vi "Manipulator Panel.vi"() -> ()   [LabVIEW 2014]
uses:
  <vilib>/Platform/TimedLoop/XDataNode/timing_clust.ctl
  <vilib>/Platform/TimedLoop/XDataNode/nitl_modes.ctl
  <vilib>/Platform/TimedLoop/XDataNode/wakeup.ctl
  <vilib>/Utility/inputDevices.llb/joystickAcquire.vi
  <vilib>/Platform/TimedLoop/XDataNode/XDataNode.xnode
  <vilib>/Platform/TimedLoop/XDataNode/XDNodeRunTimeDep.lvlib
panel:
  in  "Joystick Selector":u16(ring) items=["HID Dongle", "USB PnP Sound Device"]
  in  "Use Joystick":bool
  out "axis info":T1
  out "button info":T2
  out "Active":bool
  out "Reset":bool
  in  "TCPConRef":refnum<k5>
  out "Turning off in":dbl=10.0
  in  "Power switch\nmanipulator":bool
  in  "Arm Rotate ccw":bool
  in  "Arm Rotate cw":bool
  in  "Claw close":bool
  in  "Claw open":bool
  in  "Arm right":bool
  in  "Arm left":bool
  in  "Lower arm down":bool
  in  "Lower arm up":bool
  in  "Upper arm down":bool
  in  "Upper arm up":bool
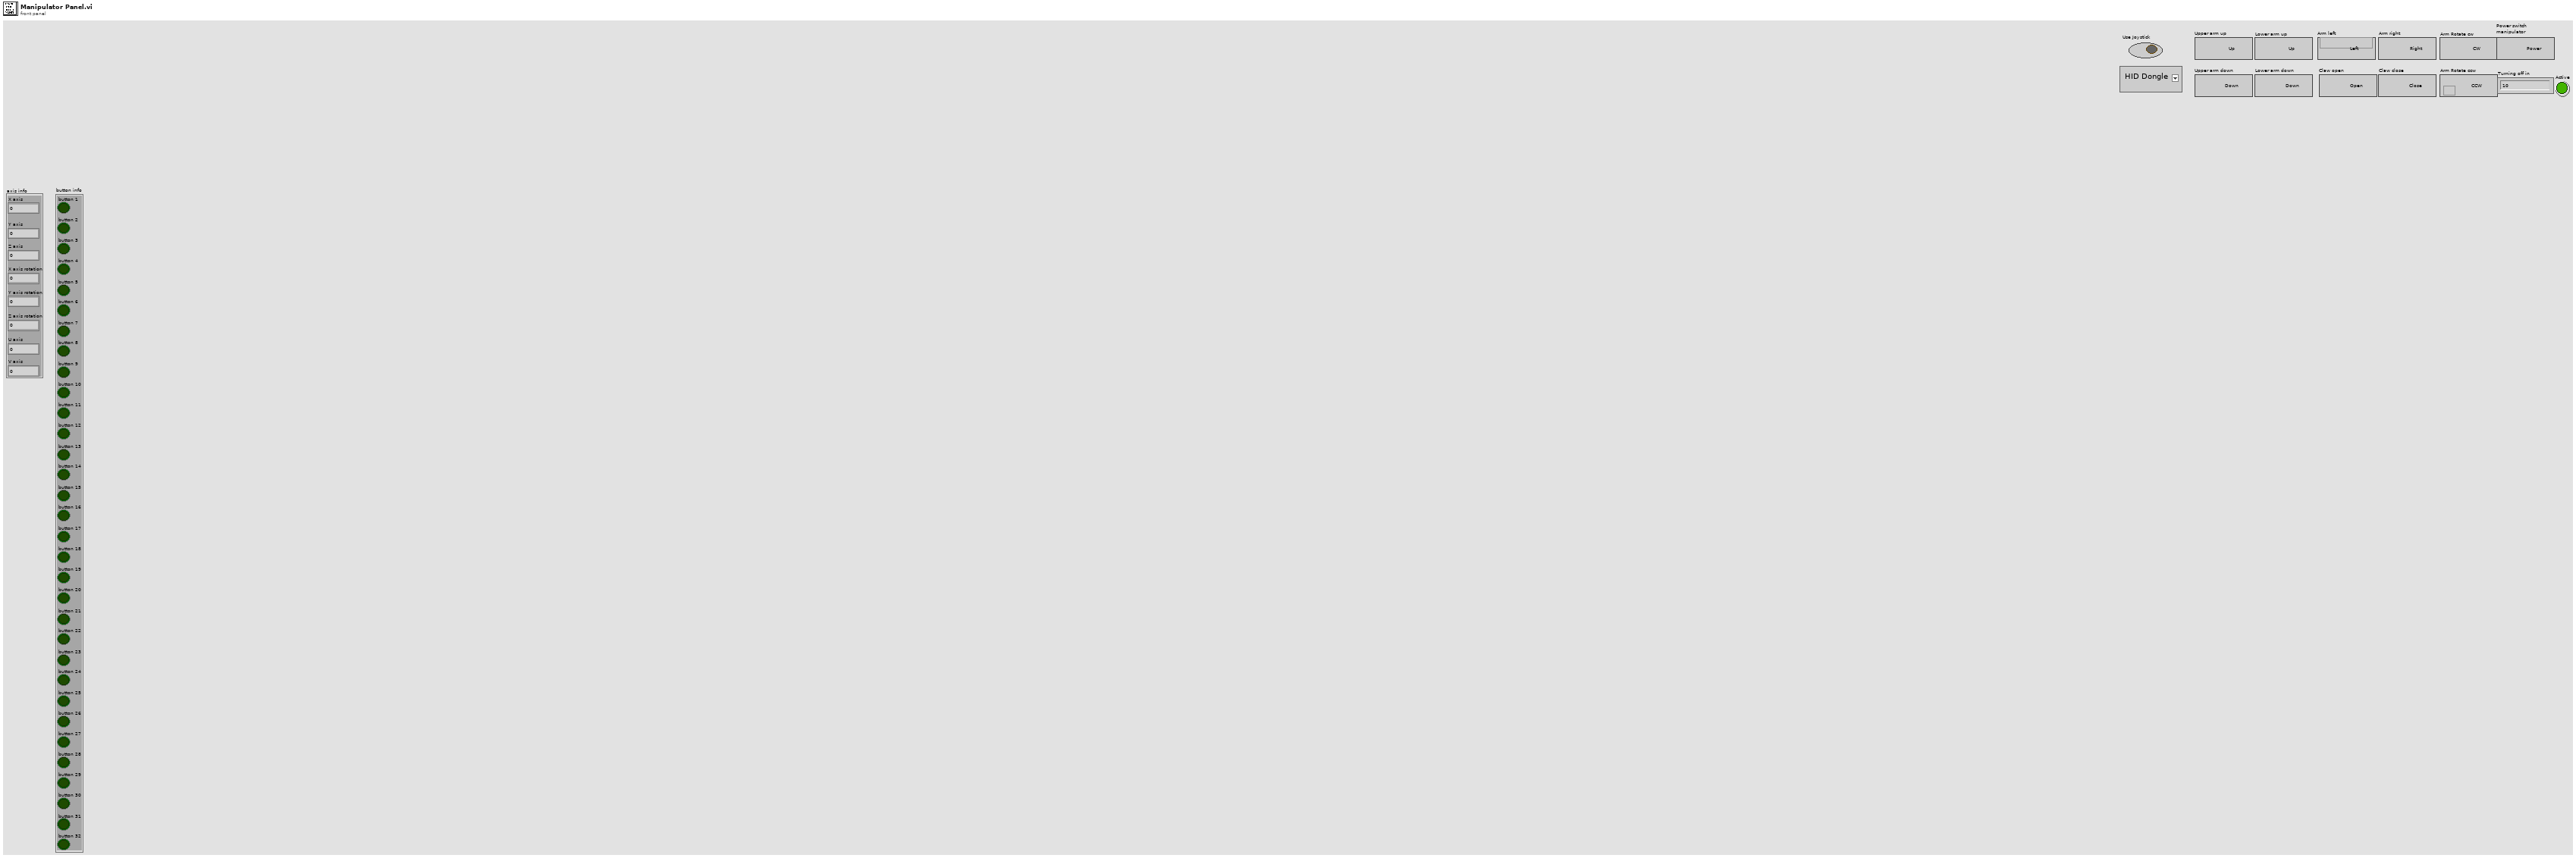
[diagram p1: front panel]
types:
  T1 = cluster{"X axis":i32, "Y axis":i32, "Z axis":i32, "X axis rotation":i32, "Y axis rotation":i32, "Z axis rotation":i32, "U axis":i32, "V axis":i32}
  T2 = cluster{"button 1":bool, "button 2":bool, "button 3":bool, "button 4":bool, "button 5":bool, "button 6":bool, "button 7":bool, "button 8":bool, "button 9":bool, "button 10":bool, "button 11":bool, "button 12":bool, "button 13":bool, "button 14":bool, "button 15":bool, "button 16":bool, "button 17":bool, "button 18":bool, "button 19":bool, "button 20":bool, "button 21":bool, "button 22":bool, "button 23":bool, "button 24":bool, "button 25":bool, "button 26":bool, "button 27":bool, "button 28":bool, "button 29":bool, "button 30":bool, "button 31":bool, "button 32":bool}
  T3 = typedef "XDNodeRunTimeDep.lvlib/timing_clust.ctl" = cluster{"Expected End [f-1]":u64, "Actual End [f-1]":u64, "Finished Late? [f-1]":bool, "Expected End [i-1]":u64, "Actual End [i-1]":u64, "Finished Late? [i-1]":bool, "Expected Start [i]":u64, "Actual Start [i]":u64, "Expected Start [f]":u64, "Actual Start [f]":u64, "Source Name":string, "Structure Name":string, "Period":i64, "Deadline":i64, "Offset":i64, "Start":i64, "Priority":i32, "Timeout":i32, "Mode":T4, "Wakeup Reason":T5, "Error":errorcluster, "Source Type":string, "Secondary Source Type":string, "Global End Time":u64, "Global Start Time":u64, "Frame Duration":u64, "Iteration Duration":u64, "Assigned CPU":i32, "I/O Scan Engine Mode":u32}
  T4 = typedef "XDNodeRunTimeDep.lvlib/nitl_modes.ctl" = enum32{"No Change", "Process missed periods, maintain original phase", "Discard missed periods, maintain original phase", "Process missed periods, ignore original phase", "Discard missed periods, ignore original phase"}
  T5 = typedef "XDNodeRunTimeDep.lvlib/wakeup.ctl" = enum32{"Normal", "Aborted", "Asynchronous wakeup", "Timing source error", "Timed loop error", "Timeout"}
  T6 = cluster{"axes total":u32, "buttons total":u32, "pov total":u32, "device name":string}[]
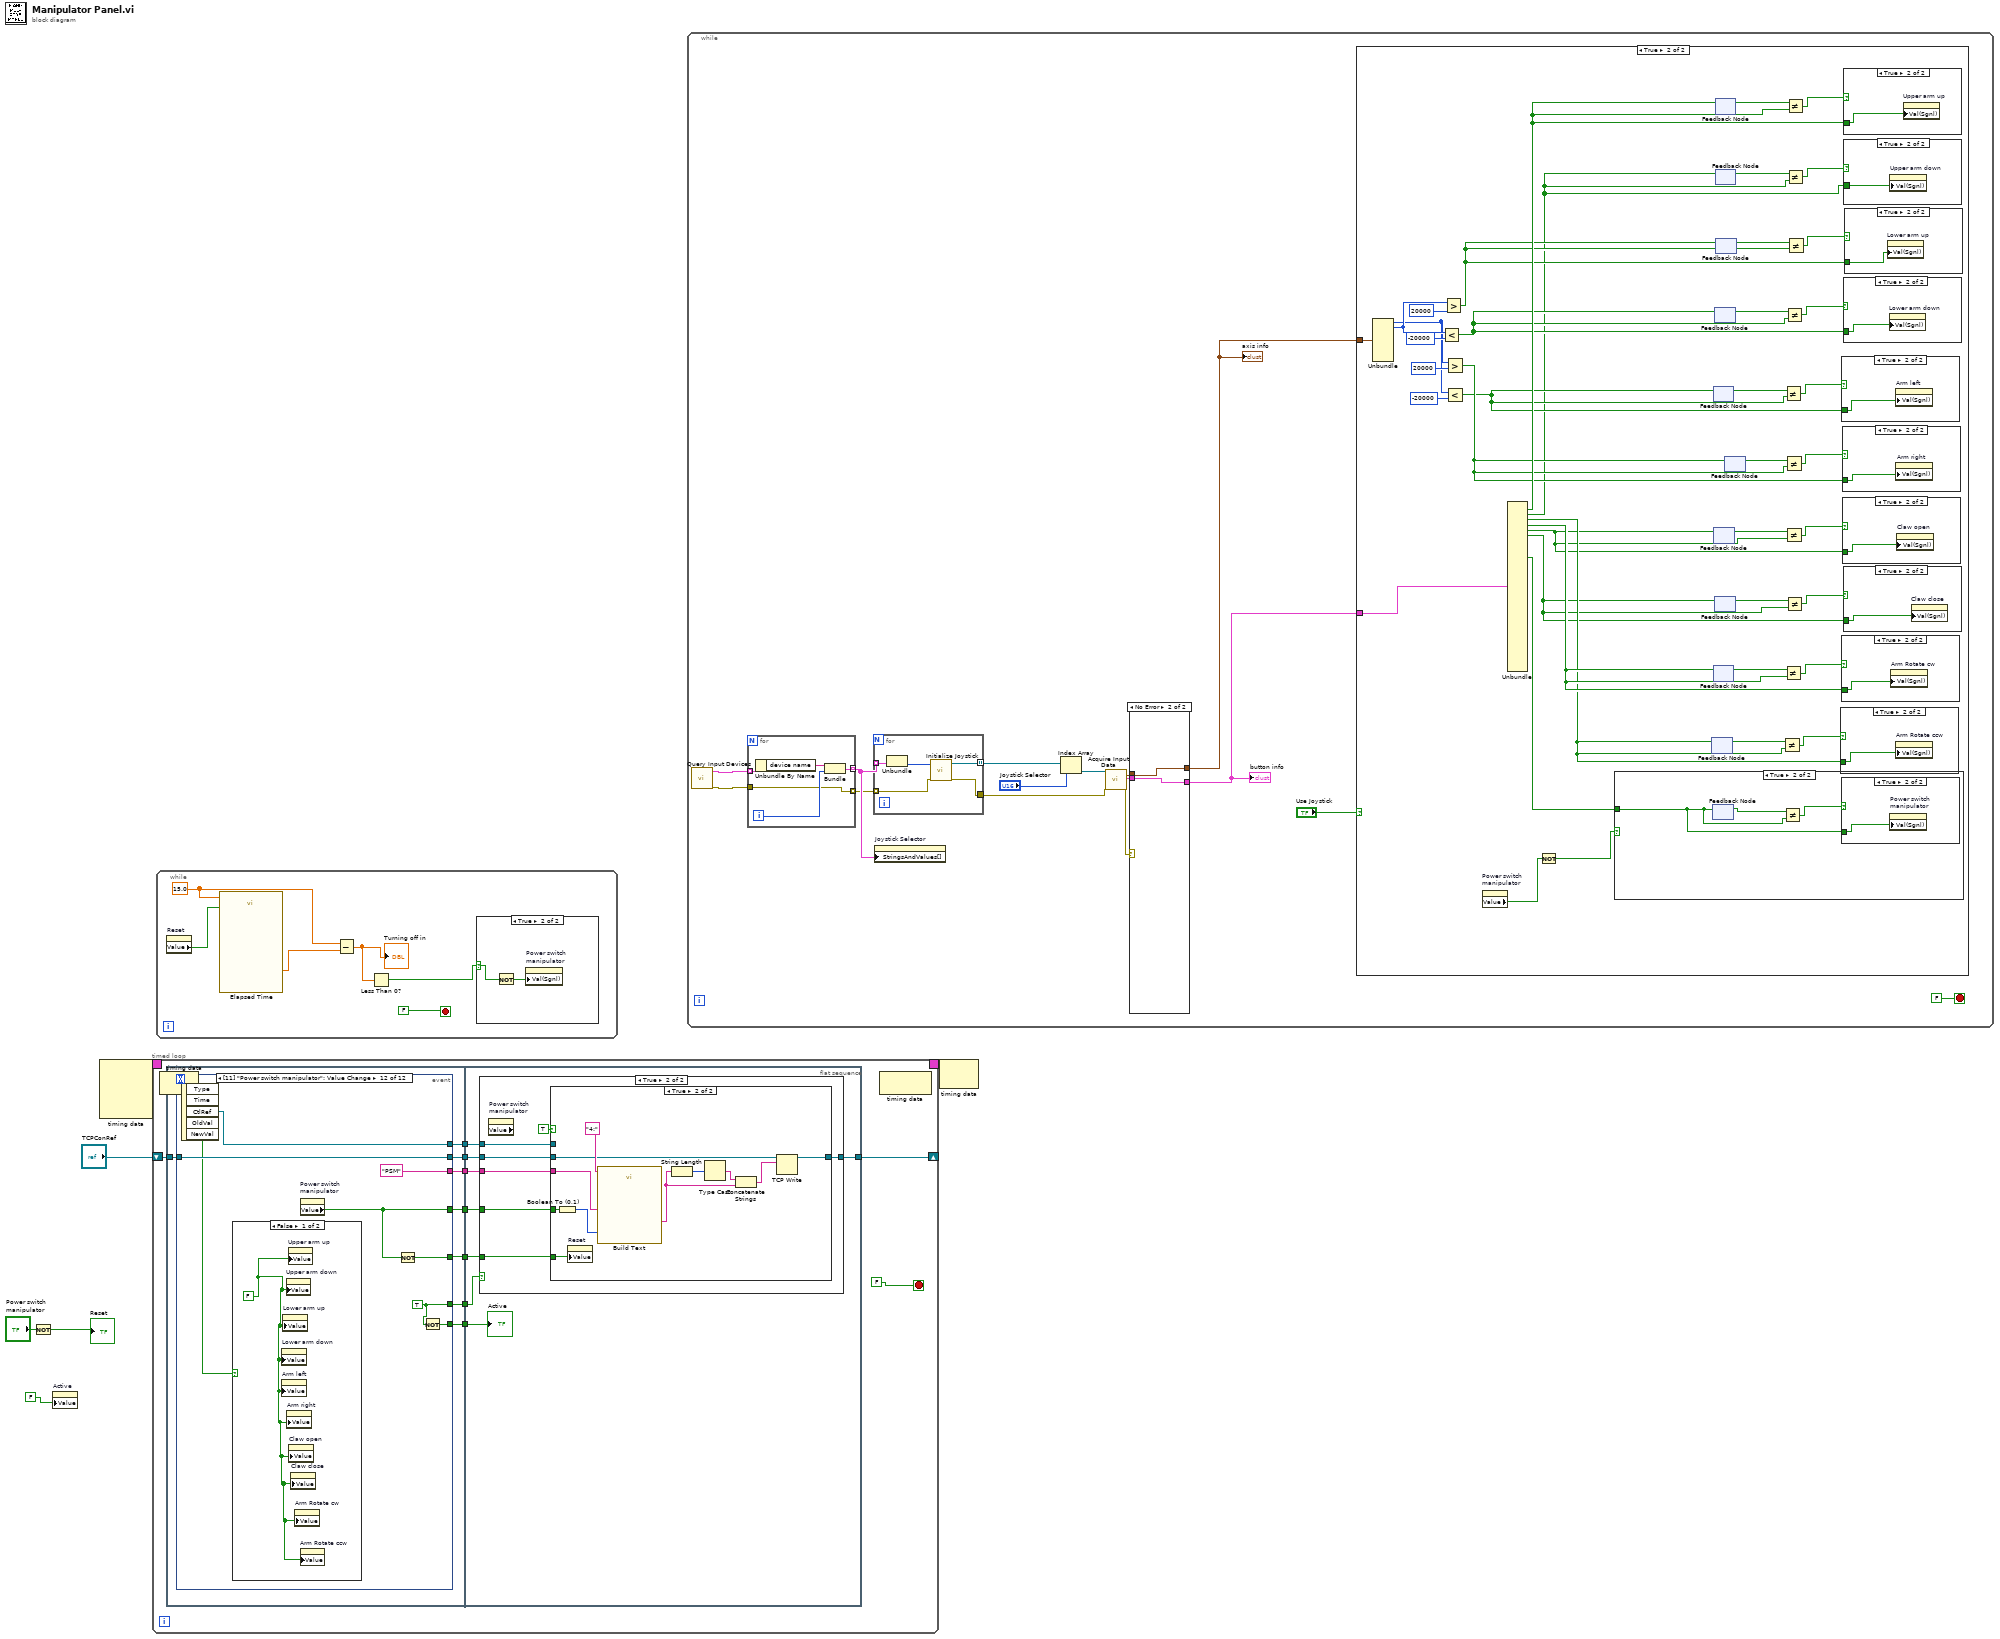
[diagram p0: block diagram]
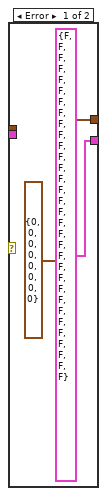
[diagram p2: hidden frame]
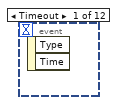
[diagram p16: hidden frame]
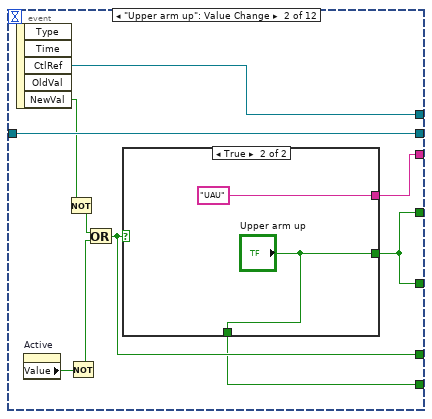
[diagram p17: hidden frame]
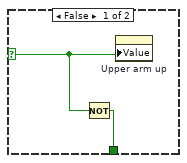
[diagram p18: hidden frame]
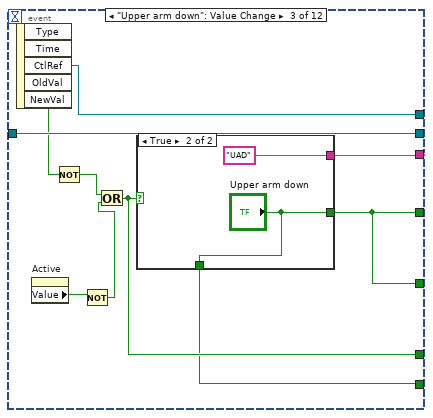
[diagram p19: hidden frame]
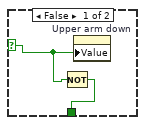
[diagram p20: hidden frame]
diagram:
  n1 = Not(x="Power switch\nmanipulator") -> (.not. x?=→"Reset":bool)
  n2 = property on="Active" class="Bool (strict)"("Value"=FALSE) -> ()  [unwired: 2 in, 2 out]
  n3 = node-c288() -> (w2:T3)  [unwired: 4 in]
  n4 = timed-loop {
    shift-right: [w9] -> _
    shift-left: "TCPConRef" -> [w15]
    timing: w2 -> [_]
    timing-out: [_] -> w1
    stop <- FALSE stop-if-true
    n5 = node-c288() -> ()  [unwired: 1 in, 1 out]
    n6 = flat-sequence {
      tunnel: w15 -> [w26]
      tunnel: [w25] -> w14
      tunnel: [w24] -> w13
      tunnel: [w23] -> w12
      tunnel: [w22] -> w11
      tunnel: [w21] -> w10
      tunnel: [w20] -> w8
      tunnel: [w19] -> w7
      tunnel: w14 -> [w182]
      tunnel: w13 -> [w181]
      tunnel: w12 -> [w180]
      tunnel: w11 -> [w183]
      tunnel: w10 -> [w179]
      tunnel: [w178] -> w9
      tunnel: w8 -> [w177]
      tunnel: w7 -> [w176]
      frame #0 {
        n7 = event shown="[11] \"Power switch manipulator\": Value Change" {
          selector: _ -> [_ _ _ _ _ _ _ _ _ _ _ _]
          dyn-events: _ -> [_ _ _ _ _ _ _ _ _ _ _ _]
          timeout: _ -> [_ _ _ _ _ _ _ _ _ _ _ _]
          tunnel: w26 -> [_ w36 w49 w63 w76 w92 w104 w119 w133 w146 w160 w173]
          tunnel: [_ w36 w49 w63 w76 w92 w104 w119 w133 w146 w160 w173] -> w25
          tunnel: [_ w30 w50 w62 w78 w91 w105 w120 w134 w147 w161 "PSM"] -> w24
          tunnel: [_ w29 w47 w64 w77 w90 w106 w117 w131 w148 w162 w171] -> w23
          tunnel: [_ w29 w47 w64 w77 w90 w106 w117 w131 w148 w162 w172] -> w21
          tunnel: [_ w35 w48 w61 w75 w89 w103 w118 w132 w145 w159 w170] -> w22
          tunnel: [_ w28 w42 w56 w70 w84 w98 w112 w126 w140 w154 w167] -> w20
          tunnel: [_ w27 w41 w55 w69 w83 w97 w111 w125 w139 w153 w168] -> w19
          event Timeout {
            n8 = event-data() -> ()  [unwired: 1 in, 2 out]
          }
          event "Upper arm up": Value Change {
            n9 = event-data() -> ("CtlRef"=w35:refnum<vi>, "NewVal"=w34:bool)  [unwired: 1 in, 3 out]
            n10 = property on="Active" class="Bool (strict)"() -> ("Value"=w33:bool)  [unwired: 2 in, 2 out]
            n11 = Not(x=w34) -> (.not. x?=w31:bool)
            n12 = Not(x=w33) -> (.not. x?=w32:bool)
            n13 = Or(x=w31, y=w32) -> (x .or. y?=w28:bool)
            n14 = case shown="True" w28 {
              selector: w28 -> [w38 _]
              tunnel: [_ "UAU"] -> w30
              tunnel: [_ "Upper arm up"] -> w29
              tunnel: [w37 "Upper arm up"] -> w27
              frame False {
                n15 = Not(x=w38) -> (.not. x?=w37:bool)
                n16 = property on="Upper arm up" class="Bool (strict)"("Value"=w38) -> ()  [unwired: 2 in, 2 out]
              }
              frame True {
              }
            }
          }
          event "Upper arm down": Value Change {
            n17 = event-data() -> ("CtlRef"=w48:refnum<vi>, "NewVal"=w43:bool)  [unwired: 1 in, 3 out]
            n18 = property on="Active" class="Bool (strict)"() -> ("Value"=w46:bool)  [unwired: 2 in, 2 out]
            n19 = Not(x=w43) -> (.not. x?=w44:bool)
            n20 = Not(x=w46) -> (.not. x?=w45:bool)
            n21 = Or(x=w44, y=w45) -> (x .or. y?=w42:bool)
            n22 = case shown="True" w42 {
              selector: w42 -> [w52 _]
              tunnel: [_ "UAD"] -> w50
              tunnel: [_ "Upper arm down"] -> w47
              tunnel: [w51 "Upper arm down"] -> w41
              frame False {
                n23 = Not(x=w52) -> (.not. x?=w51:bool)
                n24 = property on="Upper arm down" class="Bool (strict)"("Value"=w52) -> ()  [unwired: 2 in, 2 out]
              }
              frame True {
              }
            }
          }
          event "Lower arm up": Value Change {
            n25 = event-data() -> ("CtlRef"=w61:refnum<vi>, "NewVal"=w60:bool)  [unwired: 1 in, 3 out]
            n26 = property on="Active" class="Bool (strict)"() -> ("Value"=w57:bool)  [unwired: 2 in, 2 out]
            n27 = Not(x=w60) -> (.not. x?=w59:bool)
            n28 = Not(x=w57) -> (.not. x?=w58:bool)
            n29 = Or(x=w59, y=w58) -> (x .or. y?=w56:bool)
            n30 = case shown="True" w56 {
              selector: w56 -> [w66 _]
              tunnel: [_ "Lower arm up"] -> w64
              tunnel: [_ "LAU"] -> w62
              tunnel: [w65 "Lower arm up"] -> w55
              frame False {
                n31 = Not(x=w66) -> (.not. x?=w65:bool)
                n32 = property on="Lower arm up" class="Bool (strict)"("Value"=w66) -> ()  [unwired: 2 in, 2 out]
              }
              frame True {
              }
            }
          }
          event "Lower arm down": Value Change {
            n33 = event-data() -> ("CtlRef"=w75:refnum<vi>, "NewVal"=w71:bool)  [unwired: 1 in, 3 out]
            n34 = property on="Active" class="Bool (strict)"() -> ("Value"=w74:bool)  [unwired: 2 in, 2 out]
            n35 = Not(x=w71) -> (.not. x?=w72:bool)
            n36 = Not(x=w74) -> (.not. x?=w73:bool)
            n37 = Or(x=w72, y=w73) -> (x .or. y?=w70:bool)
            n38 = case shown="False" w70 {
              selector: w70 -> [w79 _]
              tunnel: [_ "LAD"] -> w78
              tunnel: [_ "Lower arm down"] -> w77
              tunnel: [w80 "Lower arm down"] -> w69
              frame False {
                n39 = property on="Lower arm down" class="Bool (strict)"("Value"=w79) -> ()  [unwired: 2 in, 2 out]
                n40 = Not(x=w79) -> (.not. x?=w80:bool)
              }
              frame True {
              }
            }
          }
          event "Arm left": Value Change {
            n41 = event-data() -> ("CtlRef"=w89:refnum<vi>, "NewVal"=w87:bool)  [unwired: 1 in, 3 out]
            n42 = property on="Active" class="Bool (strict)"() -> ("Value"=w88:bool)  [unwired: 2 in, 2 out]
            n43 = Not(x=w87) -> (.not. x?=w86:bool)
            n44 = Not(x=w88) -> (.not. x?=w85:bool)
            n45 = Or(x=w86, y=w85) -> (x .or. y?=w84:bool)
            n46 = case shown="True" w84 {
              selector: w84 -> [w94 _]
              tunnel: [_ "MAL"] -> w91
              tunnel: [_ "Arm left"] -> w90
              tunnel: [w93 "Arm left"] -> w83
              frame False {
                n47 = Not(x=w94) -> (.not. x?=w93:bool)
                n48 = property on="Arm left" class="Bool (strict)"("Value"=w94) -> ()  [unwired: 2 in, 2 out]
              }
              frame True {
              }
            }
          }
          event "Arm right": Value Change {
            n49 = event-data() -> ("CtlRef"=w103:refnum<vi>, "NewVal"=w100:bool)  [unwired: 1 in, 3 out]
            n50 = property on="Active" class="Bool (strict)"() -> ("Value"=w99:bool)  [unwired: 2 in, 2 out]
            n51 = Not(x=w100) -> (.not. x?=w101:bool)
            n52 = Not(x=w99) -> (.not. x?=w102:bool)
            n53 = Or(x=w101, y=w102) -> (x .or. y?=w98:bool)
            n54 = case shown="True" w98 {
              selector: w98 -> [w108 _]
              tunnel: [_ "Arm right"] -> w106
              tunnel: [_ "MAR"] -> w105
              tunnel: [w107 "Arm right"] -> w97
              frame False {
                n55 = Not(x=w108) -> (.not. x?=w107:bool)
                n56 = property on="Arm right" class="Bool (strict)"("Value"=w108) -> ()  [unwired: 2 in, 2 out]
              }
              frame True {
              }
            }
          }
          event "Claw open": Value Change {
            n57 = event-data() -> ("CtlRef"=w118:refnum<vi>, "NewVal"=w116:bool)  [unwired: 1 in, 3 out]
            n58 = property on="Active" class="Bool (strict)"() -> ("Value"=w113:bool)  [unwired: 2 in, 2 out]
            n59 = Not(x=w116) -> (.not. x?=w115:bool)
            n60 = Not(x=w113) -> (.not. x?=w114:bool)
            n61 = Or(x=w115, y=w114) -> (x .or. y?=w112:bool)
            n62 = case shown="True" w112 {
              selector: w112 -> [w121 _]
              tunnel: [_ "CLO"] -> w120
              tunnel: [_ "Claw open"] -> w117
              tunnel: [w122 "Claw open"] -> w111
              frame False {
                n63 = Not(x=w121) -> (.not. x?=w122:bool)
                n64 = property on="Claw open" class="Bool (strict)"("Value"=w121) -> ()  [unwired: 2 in, 2 out]
              }
              frame True {
              }
            }
          }
          event "Claw close": Value Change {
            n65 = event-data() -> ("CtlRef"=w132:refnum<vi>, "NewVal"=w127:bool)  [unwired: 1 in, 3 out]
            n66 = property on="Active" class="Bool (strict)"() -> ("Value"=w128:bool)  [unwired: 2 in, 2 out]
            n67 = Not(x=w127) -> (.not. x?=w130:bool)
            n68 = Not(x=w128) -> (.not. x?=w129:bool)
            n69 = Or(x=w130, y=w129) -> (x .or. y?=w126:bool)
            n70 = case shown="True" w126 {
              selector: w126 -> [w136 _]
              tunnel: [_ "CLC"] -> w134
              tunnel: [_ "Claw close"] -> w131
              tunnel: [w135 "Claw close"] -> w125
              frame False {
                n71 = Not(x=w136) -> (.not. x?=w135:bool)
                n72 = property on="Claw close" class="Bool (strict)"("Value"=w136) -> ()  [unwired: 2 in, 2 out]
              }
              frame True {
              }
            }
          }
          event "Arm Rotate cw": Value Change {
            n73 = event-data() -> ("CtlRef"=w145:refnum<vi>, "NewVal"=w142:bool)  [unwired: 1 in, 3 out]
            n74 = property on="Active" class="Bool (strict)"() -> ("Value"=w141:bool)  [unwired: 2 in, 2 out]
            n75 = Not(x=w142) -> (.not. x?=w143:bool)
            n76 = Not(x=w141) -> (.not. x?=w144:bool)
            n77 = Or(x=w143, y=w144) -> (x .or. y?=w140:bool)
            n78 = case shown="True" w140 {
              selector: w140 -> [w150 _]
              tunnel: [_ "Arm Rotate cw"] -> w148
              tunnel: [_ "ARR"] -> w147
              tunnel: [w149 "Arm Rotate cw"] -> w139
              frame False {
                n79 = Not(x=w150) -> (.not. x?=w149:bool)
                n80 = property on="Arm Rotate cw" class="Bool (strict)"("Value"=w150) -> ()  [unwired: 2 in, 2 out]
              }
              frame True {
              }
            }
          }
          event "Arm Rotate ccw": Value Change {
            n81 = event-data() -> ("CtlRef"=w159:refnum<vi>, "NewVal"=w156:bool)  [unwired: 1 in, 3 out]
            n82 = property on="Active" class="Bool (strict)"() -> ("Value"=w155:bool)  [unwired: 2 in, 2 out]
            n83 = Not(x=w156) -> (.not. x?=w157:bool)
            n84 = Not(x=w155) -> (.not. x?=w158:bool)
            n85 = Or(x=w157, y=w158) -> (x .or. y?=w154:bool)
            n86 = case shown="True" w154 {
              selector: w154 -> [w164 _]
              tunnel: [_ "Arm Rotate ccw"] -> w162
              tunnel: [_ "ARL"] -> w161
              tunnel: [w163 "Arm Rotate ccw"] -> w153
              frame False {
                n87 = Not(x=w164) -> (.not. x?=w163:bool)
                n88 = property on="Arm Rotate ccw" class="Bool (strict)"("Value"=w164) -> ()  [unwired: 2 in, 2 out]
              }
              frame True {
              }
            }
          }
          event "Power switch\nmanipulator": Value Change {
            w167 = TRUE
            n89 = event-data() -> ("CtlRef"=w170:refnum<vi>, "NewVal"=w169:bool)  [unwired: 1 in, 3 out]
            n90 = case shown="False" w169 {
              frame False {
                w175 = FALSE
                n91 = property on="Lower arm down" class="Bool (strict)"("Value"=w175) -> ()  [unwired: 2 in, 2 out]
                n92 = property on="Arm left" class="Bool (strict)"("Value"=w175) -> ()  [unwired: 2 in, 2 out]
                n93 = property on="Lower arm up" class="Bool (strict)"("Value"=w175) -> ()  [unwired: 2 in, 2 out]
                n94 = property on="Upper arm down" class="Bool (strict)"("Value"=w175) -> ()  [unwired: 2 in, 2 out]
                n95 = property on="Arm right" class="Bool (strict)"("Value"=w175) -> ()  [unwired: 2 in, 2 out]
                n96 = property on="Upper arm up" class="Bool (strict)"("Value"=w175) -> ()  [unwired: 2 in, 2 out]
                n97 = property on="Claw open" class="Bool (strict)"("Value"=w175) -> ()  [unwired: 2 in, 2 out]
                n98 = property on="Claw close" class="Bool (strict)"("Value"=w175) -> ()  [unwired: 2 in, 2 out]
                n99 = property on="Arm Rotate cw" class="Bool (strict)"("Value"=w175) -> ()  [unwired: 2 in, 2 out]
                n100 = property on="Arm Rotate ccw" class="Bool (strict)"("Value"=w175) -> ()  [unwired: 2 in, 2 out]
              }
              frame True {
              }
            }
            n101 = property on="Power switch\nmanipulator" class="Bool (strict)"() -> ("Value"=w171:bool)  [unwired: 2 in, 2 out]
            n102 = Not(x=w171) -> (.not. x?=w172:bool)
            n103 = Not(x=w167) -> (.not. x?=w168:bool)
          }
        }
      }
      frame #1 {
        n104 = case shown="True" w177 {
          tunnel: w183 -> [_ w191]
          tunnel: w182 -> [w184 w190]
          tunnel: w181 -> [_ w189]
          tunnel: w180 -> [_ w188]
          tunnel: w179 -> [_ w187]
          tunnel: [w184 w186] -> w178
          frame False {
          }
          frame True {
            n105 = property on="Power switch\nmanipulator" class="Bool (strict)" props=["Value"]() -> ()  [unwired: 2 in, 3 out]
            n106 = case shown="True" TRUE {
              tunnel: w190 -> [w193 w204]
              tunnel: [w193 w203] -> w186
              tunnel: w189 -> [_ w212]
              tunnel: w188 -> [_ w207]
              tunnel: w191 -> [w194 _]
              tunnel: w187 -> [_ w205]
              frame False {
                n107 = control-ref of="Power switch\nmanipulator"() -> (w195:refnum<vi>)
                n108 = Not Equal?(x=w194, y=w195) -> (x != y?=w192:bool)
                n109 = case shown="True" w192 {
                  tunnel: w194 -> [w198 w200]
                  frame False {
                    n110 = property class="Bool (strict)"(reference=w198) -> ("Value"=w197:bool)  [unwired: 1 in, 2 out]
                    n111 = Not(x=w197) -> (.not. x?=w196:bool)
                    n112 = property on="Reset" class="Bool (strict)"("Value"=w196) -> ()  [unwired: 2 in, 2 out]
                  }
                  frame True {
                    n113 = property class="Bool (strict)"(reference=w200, "Value"=FALSE) -> ()  [unwired: 1 in, 2 out]
                    n114 = One Button Dialog(message="You must start the\nmanipulator engine first") -> ()  [unwired: 1 in, 1 out]
                  }
                }
              }
              frame True {
                n115 = Boolean To (0,1)(Boolean=w207) -> (0, 1=w206:i16)
                n116 = property on="Reset" class="Bool (strict)"("Value"=w205) -> ()  [unwired: 2 in, 2 out]
                n117 = call "Build Text"("Beginning Text"="4:", "ControlID"=w212, "Bool"=w206) -> ("Result"=w208:string)  [unwired: 11 in, 1 out]
                n118 = String Length(string=w208) -> (length=w210:i32)
                n119 = Type Cast(x=w210) -> (*(type *) &x=w209:string)  [unwired: 1 in]
                n120 = Concatenate Strings(w209, w208) -> (w202:string)
                n121 = TCP Write(connection ID=w204, data in=w202) -> (connection ID out=w203:refnum<k5>)  [unwired: 2 in, 2 out]
              }
            }
          }
        }
        "Active" <- w176
      }
    }
    n122 = node-c288() -> ()  [unwired: 1 in, 1 out]
  }
  n123 = while {
    stop <- FALSE stop-if-true
    w218 = 15.0
    n124 = property on="Reset" class="Bool (strict)"() -> ("Value"=w215:bool)  [unwired: 2 in, 2 out]
    n125 = call "Elapsed Time"("Time Target (s)"=w218, "Reset"=w215) -> ("Elapsed Time (s)"=w217:dbl)  [unwired: 10 in, 7 out]
    n126 = Subtract(x=w218, y=w217) -> (x-y=w214:dbl)
    "Turning off in" <- w214
    n127 = Less Than 0?(x=w214) -> (x < 0?=w213:bool)
    n128 = case shown="True" w213 {
      selector: w213 -> [_ w219]
      frame False {
      }
      frame True {
        n129 = Not(x=w219) -> (.not. x?=w220:bool)
        n130 = property on="Power switch\nmanipulator" class="Bool (strict)"("Val(Sgnl)"=w220) -> ()  [unwired: 2 in, 2 out]
      }
    }
  }
  n131 = while {
    stop <- FALSE stop-if-true
    n132 = call <vilib>:"Query Input Devices.vi"() -> ("error out"=w230:errorcluster, "joystick info"=w235:T6)  [unwired: 8 in, 2 out]
    n133 = for {
      tunnel: w235 -> [w244] mode=indexing
      tunnel: [w241] -> w229 mode=indexing
      tunnel: [w240] -> w225 mode=indexing
      tunnel: w230 -> [w240]
      i -> [w242]
      n134 = Unbundle By Name(w244) -> ("device name"=w243:string)
      n135 = Bundle("device name"=w243, w242) -> (w241:cluster{"device name":string, i32})  [unwired: 1 in]
    }
    n136 = for {
      tunnel: w229 -> [w248] mode=indexing
      tunnel: [w249] -> w226 mode=indexing
      tunnel: w225 -> [w246] mode=indexing
      tunnel: [w245] -> w221
      n137 = Unbundle(w248) -> (w247:i32)  [unwired: 1 out]
      n138 = call <vilib>:"Initialize Joystick.vi"("error in (no error)"=w246, "device index"=w247) -> ("error out"=w245:errorcluster, "device ID"=w249:refnum<k1>)  [unwired: 8 in]
    }
    n139 = property on="Joystick Selector" class="Ring (strict)"("StringsAndValues[]"=w229) -> ()  [unwired: 2 in, 2 out]
    n140 = Index Array(array=w226, index="Joystick Selector") -> (element=w227:refnum<k1>)
    n141 = call-poly <vilib>:"Acquire Input Data.vi"("device ID"=w227, "error in (no error)"=w221) -> ("axis info"=w223:T1, "button info"=w222:T2, "error out"=w224:errorcluster)  [unwired: 13 in, 2 out]
    n142 = case shown="No Error" w224 {
      tunnel: [T1 {"X axis"=0, "Y axis"=0, "Z axis"=0, "X axis rotation"=0, "Y axis rotation"=0, "Z axis rotation"=0, "U axis"=0, "V axis"=0} ("axis info") w239] -> w231
      tunnel: w223 -> [_ w239]
      tunnel: [T2 {"button 1"=FALSE, "button 2"=FALSE, "button 3"=FALSE, "button 4"=FALSE, "button 5"=FALSE, "button 6"=FALSE, "button 7"=FALSE, "button 8"=FALSE, "button 9"=FALSE, "button 10"=FALSE, "button 11"=FALSE, "button 12"=FALSE, "button 13"=FALSE, "button 14"=FALSE, "button 15"=FALSE, "button 16"=FALSE, "button 17"=FALSE, "button 18"=FALSE, "button 19"=FALSE, "button 20"=FALSE, "button 21"=FALSE, "button 22"=FALSE, "button 23"=FALSE, "button 24"=FALSE, "button 25"=FALSE, "button 26"=FALSE, "button 27"=FALSE, "button 28"=FALSE, "button 29"=FALSE, "button 30"=FALSE, "button 31"=FALSE, "button 32"=FALSE} ("button info") w238] -> w233
      tunnel: w222 -> [_ w238]
      frame Error {
      }
      frame No Error {
      }
    }
    "axis info" <- w231
    "button info" <- w233
    n143 = case shown="True" "Use Joystick" {
      tunnel: w233 -> [_ w290]
      tunnel: w231 -> [_ w264]
      frame False {
      }
      frame True {
        n144 = Unbundle(w264) -> ("X axis"=w256:i32, "Y axis"=w261:i32)  [unwired: 6 out]
        n145 = Less?(x=w261, y=-20000) -> (x < y?=w262:bool)
        n146 = Greater?(x=w261, y=20000) -> (0:w259:bool)
        n147 = Greater?(x=w256, y=20000) -> (0:w255:bool)
        n148 = Less?(x=w256, y=-20000) -> (x < y?=w254:bool)
        n149 = property on="Power switch\nmanipulator" class="Bool (strict)"() -> ("Value"=w250:bool)  [unwired: 2 in, 2 out]
        n150 = Unbundle(w290) -> ("button 2"=w269:bool, "button 3"=w251:bool, "button 4"=w267:bool, "button 5"=w268:bool, "button 6"=w266:bool, "button 7"=w265:bool, "button 11"=w253:bool)  [unwired: 25 out]
        n151 = Not(x=w250) -> (.not. x?=w252:bool)
        n152 = case shown="True" w252 {
          tunnel: w253 -> [_ w291]
          frame False {
          }
          frame True {
            n153 = feedback #1() -> (w293:bool)  [unwired: 1 in]
            n154 = feedback-in #1(w291) -> ()
            n155 = Not Equal?(x=w293, y=w291) -> (x != y?=w292:bool)
            n156 = case shown="True" w292 {
              tunnel: w291 -> [_ w294]
              frame False {
              }
              frame True {
                n157 = property on="Power switch\nmanipulator" class="Bool (strict)"("Val(Sgnl)"=w294) -> ()  [unwired: 2 in, 2 out]
              }
            }
          }
        }
        n158 = feedback #2() -> (w282:bool)  [unwired: 1 in]
        n159 = feedback-in #2(w267) -> ()
        n160 = feedback #3() -> (w279:bool)  [unwired: 1 in]
        n161 = feedback-in #3(w254) -> ()
        n162 = feedback #4() -> (w285:bool)  [unwired: 1 in]
        n163 = feedback-in #4(w268) -> ()
        n164 = feedback-in #5(w266) -> ()
        n165 = feedback #5() -> (w289:bool)  [unwired: 1 in]
        n166 = feedback #6() -> (w276:bool)  [unwired: 1 in]
        n167 = feedback-in #6(w262) -> ()
        n168 = feedback #7() -> (w286:bool)  [unwired: 1 in]
        n169 = feedback-in #7(w265) -> ()
        n170 = feedback #8() -> (w271:bool)  [unwired: 1 in]
        n171 = feedback-in #8(w269) -> ()
        n172 = feedback #9() -> (w272:bool)  [unwired: 1 in]
        n173 = feedback-in #9(w251) -> ()
        n174 = feedback #10() -> (w275:bool)  [unwired: 1 in]
        n175 = feedback-in #10(w259) -> ()
        n176 = feedback #11() -> (w280:bool)  [unwired: 1 in]
        n177 = feedback-in #11(w255) -> ()
        n178 = Not Equal?(x=w282, y=w267) -> (x != y?=w283:bool)
        n179 = Not Equal?(x=w279, y=w254) -> (x != y?=w278:bool)
        n180 = Not Equal?(x=w285, y=w268) -> (x != y?=w284:bool)
        n181 = Not Equal?(x=w280, y=w255) -> (x != y?=w281:bool)
        n182 = Not Equal?(x=w289, y=w266) -> (x != y?=w288:bool)
        n183 = Not Equal?(x=w276, y=w262) -> (x != y?=w277:bool)
        n184 = Not Equal?(x=w286, y=w265) -> (x != y?=w287:bool)
        n185 = Not Equal?(x=w271, y=w269) -> (x != y?=w270:bool)
        n186 = Not Equal?(x=w272, y=w251) -> (x != y?=w273:bool)
        n187 = Not Equal?(x=w275, y=w259) -> (x != y?=w274:bool)
        n188 = case shown="True" w283 {
          tunnel: w267 -> [_ w301]
          frame False {
          }
          frame True {
            n189 = property on="Arm Rotate ccw" class="Bool (strict)"("Val(Sgnl)"=w301) -> ()  [unwired: 2 in, 2 out]
          }
        }
        n190 = case shown="True" w278 {
          tunnel: w254 -> [_ w297]
          frame False {
          }
          frame True {
            n191 = property on="Arm left" class="Bool (strict)"("Val(Sgnl)"=w297) -> ()  [unwired: 2 in, 2 out]
          }
        }
        n192 = case shown="True" w284 {
          tunnel: w268 -> [_ w302]
          frame False {
          }
          frame True {
            n193 = property on="Arm Rotate cw" class="Bool (strict)"("Val(Sgnl)"=w302) -> ()  [unwired: 2 in, 2 out]
          }
        }
        n194 = case shown="True" w281 {
          tunnel: w255 -> [_ w296]
          frame False {
          }
          frame True {
            n195 = property on="Arm right" class="Bool (strict)"("Val(Sgnl)"=w296) -> ()  [unwired: 2 in, 2 out]
          }
        }
        n196 = case shown="True" w288 {
          tunnel: w266 -> [_ w304]
          frame False {
          }
          frame True {
            n197 = property on="Claw open" class="Bool (strict)"("Val(Sgnl)"=w304) -> ()  [unwired: 2 in, 2 out]
          }
        }
        n198 = case shown="True" w277 {
          tunnel: w262 -> [_ w298]
          frame False {
          }
          frame True {
            n199 = property on="Lower arm down" class="Bool (strict)"("Val(Sgnl)"=w298) -> ()  [unwired: 2 in, 2 out]
          }
        }
        n200 = case shown="True" w287 {
          tunnel: w265 -> [_ w303]
          frame False {
          }
          frame True {
            n201 = property on="Claw close" class="Bool (strict)"("Val(Sgnl)"=w303) -> ()  [unwired: 2 in, 2 out]
          }
        }
        n202 = case shown="True" w270 {
          tunnel: w269 -> [_ w295]
          frame False {
          }
          frame True {
            n203 = property on="Upper arm up" class="Bool (strict)"("Val(Sgnl)"=w295) -> ()  [unwired: 2 in, 2 out]
          }
        }
        n204 = case shown="True" w273 {
          tunnel: w251 -> [_ w300]
          frame False {
          }
          frame True {
            n205 = property on="Upper arm down" class="Bool (strict)"("Val(Sgnl)"=w300) -> ()  [unwired: 2 in, 2 out]
          }
        }
        n206 = case shown="True" w274 {
          tunnel: w259 -> [_ w299]
          frame False {
          }
          frame True {
            n207 = property on="Lower arm up" class="Bool (strict)"("Val(Sgnl)"=w299) -> ()  [unwired: 2 in, 2 out]
          }
        }
      }
    }
  }
  n208 = node-c288(w1) -> ()  [unwired: 1 out]
